vi "Configure Pattern.vi"(8 "Pattern Label":string, 9 "Pattern":string, 11 "File Dialog in":refnum<class "File Dialog.lvclass">) -> (3 "File Dialog out":refnum<class "File Dialog.lvclass">)   [LabVIEW 2018, in "File Dialog Actor.lvlib" / "File Dialog.lvclass"]
uses:
  File Dialog.lvclass
  File Dialog.lvclass/File Dialog.ctl
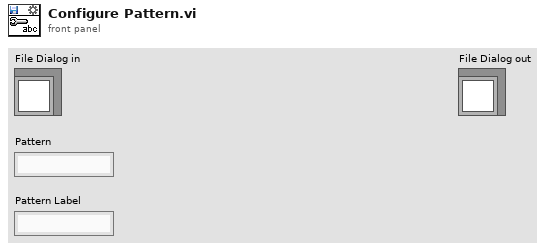
[diagram p1: front panel]
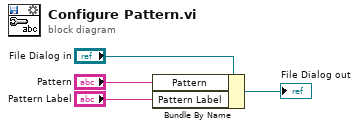
[diagram p0: block diagram]
diagram:
  n1 = Bundle By Name(cluster="File Dialog in", "Pattern"="Pattern", "Pattern Label"="Pattern Label") -> (→"File Dialog out":refnum<class "File Dialog.lvclass">)
